vi "MacroBasher_v2.vi"(4 "Changes":bool[][](array[boolean]), 5 "Path tag":string, 6 "Total time (s)":dbl, 7 "Instructions":T1 {"Steps" min=1 max=100000 step=1; "Duration" min=0.001 step=0.001 format="%_6p"}, 9 "Macro Description":string, 10 "Variable Cluster":T3 {"Variable Type" items=["Duration (s)", "Voltage (V)", "Parameter"]; "Final Val" format="%_6p"; "First Val" format="%_6p"; "Values" format="%_6p"}, 11 "Save/Open Path":path) -> ()   [LabVIEW 2018]
uses:
  Executor Files/VariableScan_Cluster.ctl
  Instructions.ctl
  Executor Files/RT/Instruction.ctl
  MacroSaveCluster.ctl
  <vilib>/Analysis/1siggen.llb/Ramp Pattern by Samples.vi
  <vilib>/Analysis/NI_AALBase.lvlib
panel:
  # "0        2       4       6        8      10     12     14     16     18      20    22     24     26     28     30     32     34     36"
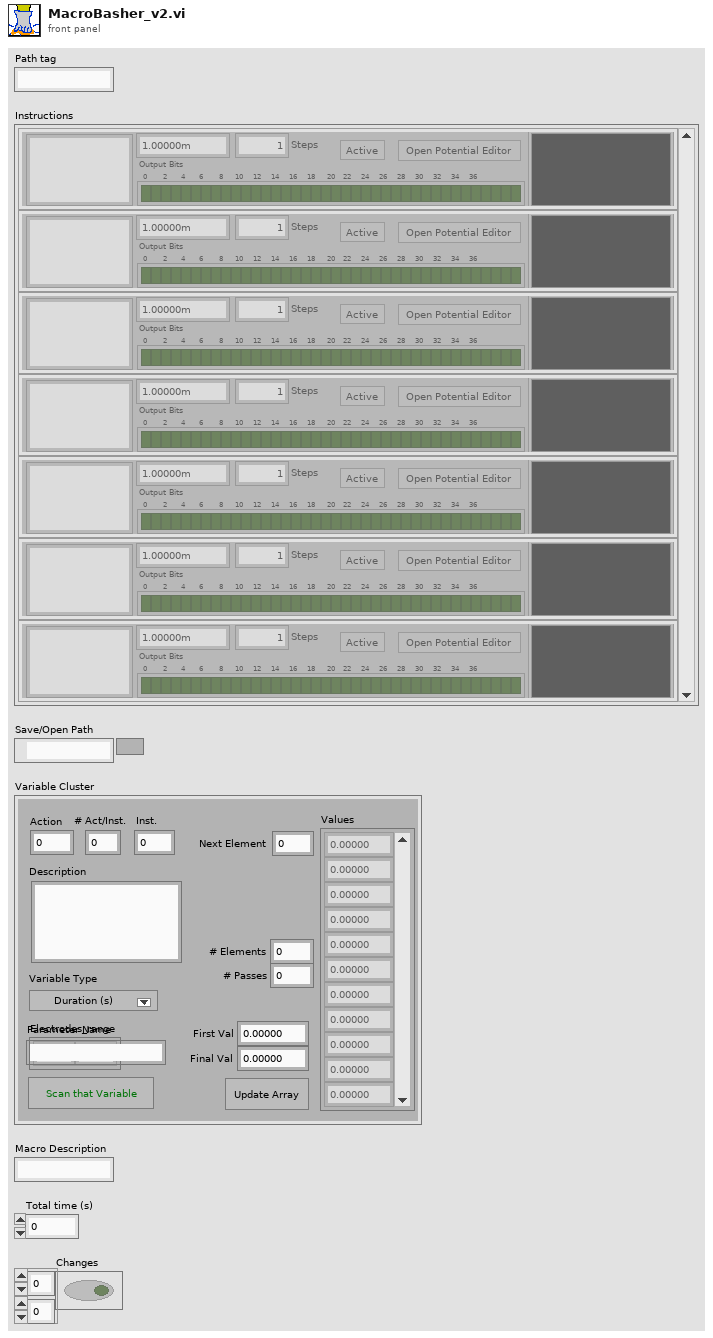
[diagram p1: front panel]
types:
  T1 = typedef "Instructions.ctl" = T2[]
  T2 = typedef "Instruction.ctl" = cluster{"Duration":dbl, "Comment":string, "Steps":i32, "Edit Potential":bool, "Output Bits":bool[], "Macro Path":path, "Potentials":dbl[], "Inherit?":bool}
  T3 = typedef "VariableScan_Cluster.ctl" = cluster{"Values":dbl[], "Action":i32, "Inst.":i32, "# Elements":i32, "Next Element":i32, "First Val":dbl, "Final Val":dbl, "Update Array":bool, "Description":string, "Variable Type":u16, "Scan Now":bool, "# Act/Inst.":i32, "Electrodes_range":i32[], "Parameter Name":string, "# Passes":i32}
  T4 = typedef "MacroSaveCluster.ctl" = cluster{"Instructions":T1, "Changes":bool[][], "Macro Description":string, "Total Time (s)":dbl, "Samples per sec":dbl}
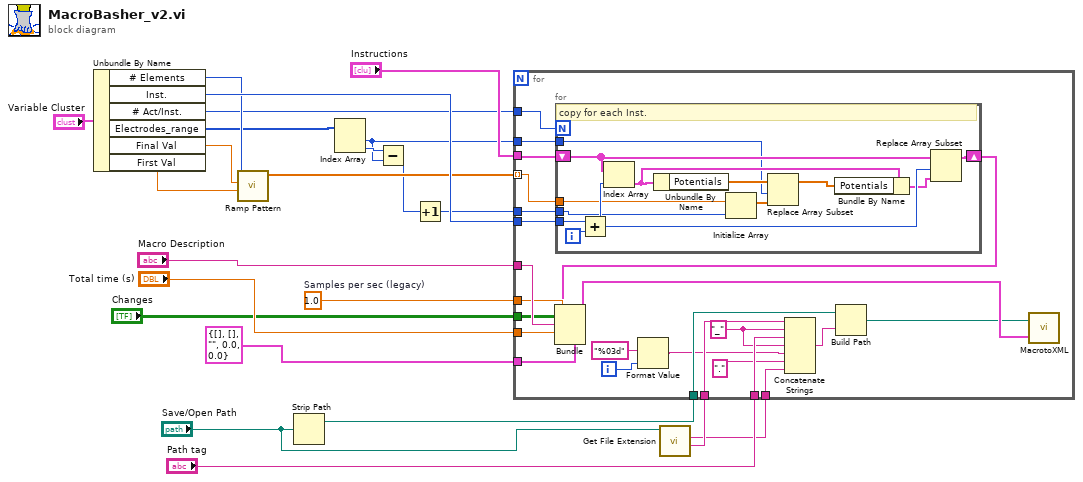
[diagram p0: block diagram]
diagram:
  w15 = 1.0  # Samples per sec (legacy)
  n1 = Unbundle By Name("Variable Cluster") -> ("# Elements"=w18:i32, "Inst."=w20:i32, "# Act/Inst."=w3:i32, "Electrodes_range"=w4:i32[], "Final Val"=w16:dbl, "First Val"=w17:dbl)
  n2 = call-poly <vilib>:"Ramp Pattern.vi"("start"=w17, "end"=w16, "samples"=w18) -> ("Ramp Pattern"=w19:dbl[])  [unwired: 7 in, 1 out]
  n3 = Strip Path(path="Save/Open Path") -> (stripped path=w21:path)  [unwired: 1 out]
  n4 = Index Array(array=w4) -> (element #1=w1:i32, element #2=w5:i32)  [unwired: 2 in]
  n5 = Subtract(x=w5, y=w1) -> (x-y=w6:i32)
  n6 = Increment(x=w6) -> (x+1=w2:i32)
  n7 = call <vilib>:"Get File Extension.vi"("file"="Save/Open Path") -> ("filename without extension"=w22:string, "lowercase file extension"=w8:string)  [unwired: 6 in, 3 out]
  n8 = for {
    tunnel: "Instructions" -> [w40]
    tunnel: "Macro Description" -> [w47]
    tunnel: "Changes" -> [w46]
    tunnel: "Total time (s)" -> [w44]
    tunnel: T4 {"Instructions"=[], "Changes"=[], "Macro Description"="", "Total Time (s)"=0.0, "Samples per sec"=0.0} ("output cluster") -> [w43]
    tunnel: w15 -> [w42]
    tunnel: w19 -> [w37] mode=indexing
    tunnel: w3 -> [w39]
    tunnel: w20 -> [w38]
    tunnel: w21 -> [w36]
    tunnel: w22 -> [w35]
    tunnel: "Path tag" -> [w34]
    tunnel: w8 -> [w29]
    tunnel: w2 -> [w25]
    tunnel: w1 -> [w24]
    i -> [w28]
    w33 = "_" ("string")
    n9 = for {
      N: w39 -> [_]
      shift-right: [w60] -> w41
      shift-left: w40 -> [w59]
      tunnel: w38 -> [w57]
      tunnel: w37 -> [w51]
      tunnel: w25 -> [w50]
      tunnel: w24 -> [w49]
      i -> [w58]
      # "copy for each Inst."
      n10 = Add(x=w57, y=w58) -> (x+y=w56:i32)
      n11 = Index Array(array=w59, index=w56) -> (element=w55:T2)
      n12 = Unbundle By Name(w55) -> ("Potentials"=w53:dbl[])
      n13 = Initialize Array(w51, w50) -> (w48:dbl[])
      n14 = Replace Array Subset(array=w53, new element=w48, index=w49) -> (w52:dbl[])
      n15 = Bundle By Name(cluster=w55, "Potentials"=w52) -> (w54:T2)
      n16 = Replace Array Subset(array=w59, new element=w54, index=w56) -> (w60:T1)
    }
    n17 = Bundle(cluster=w43, "Instructions"=w41, "Changes"=w46, "Macro Description"=w47, "Total Time (s)"=w44, "Samples per sec"=w42) -> (w45:T4)
    n18 = Format Value(format string="%03d", value (0)=w28) -> (output string=w27:string)  [unwired: 1 in]
    n19 = Concatenate Strings(w35, w33, w34, w33, w27, "." ("string"), w29) -> (w32:string)
    n20 = Build Path(base path=w36, name or relative path=w32) -> (appended path=w31:path)
    n21 = call "MacrotoXML.vi"("MacroSaveCluster"=w45, "XML File Path"=w31) -> ()  [unwired: 1 in]
  }
